vi "例3.5.vi"() -> ()   [LabVIEW 2017]
uses:
  <vilib>/regexp/Match Regular Expression.xnode
panel:
  out "数字":dbl
  out "匹配之后":string
  out "所有匹配":string
  out "匹配之前":string
  in  "字符串":string
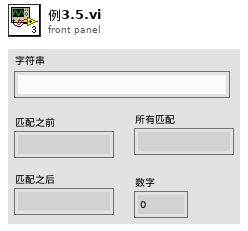
[diagram p1: front panel]
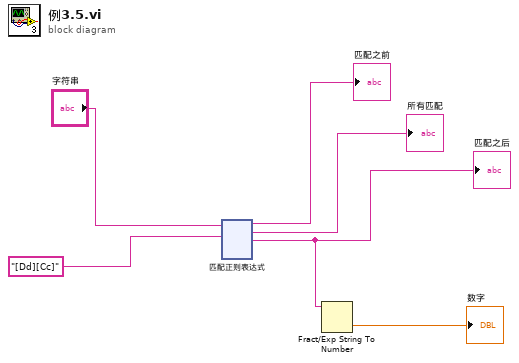
[diagram p0: block diagram]
diagram:
  n1 = xnode "匹配正则表达式"("输入字符串"="字符串", "正则表达式"="[Dd][Cc]") -> ("匹配之前"=→"匹配之前":string, "所有匹配"=→"所有匹配":string, "匹配之后"=w4:string)  [unwired: 4 in, 2 out]
  "匹配之后" <- w4
  n2 = Fract/Exp String To Number(string=w4) -> (number=→"数字":dbl)  [unwired: 3 in, 1 out]
